vi "Raw Data to Scaled Data.vi"(8 "error In":errorcluster, 9 "Data":dbl[][](array[numeric]) caption="wfm" format="%.2f", 10 "Wvf Info":T1(array[cluster]) caption="wfm info" {"reserved2" format="%.2f"; "reserved1" format="%.2f"; "offset" format="%^.3e"; "gain" format="%^.3e"; "xIncrement" format="%^.3e"; "relativeInitialX" format="%^.3e"; "absoluteInitialX" format="%^.3e"}) -> (0 "error out":errorcluster, 1 "Scaled Current":dbl[](graph), 2 "Scaled Voltage":dbl[](graph), 4 "Raw Current":dbl[](graph), 5 "Raw Voltage":dbl[](graph))   [LabVIEW 2018]
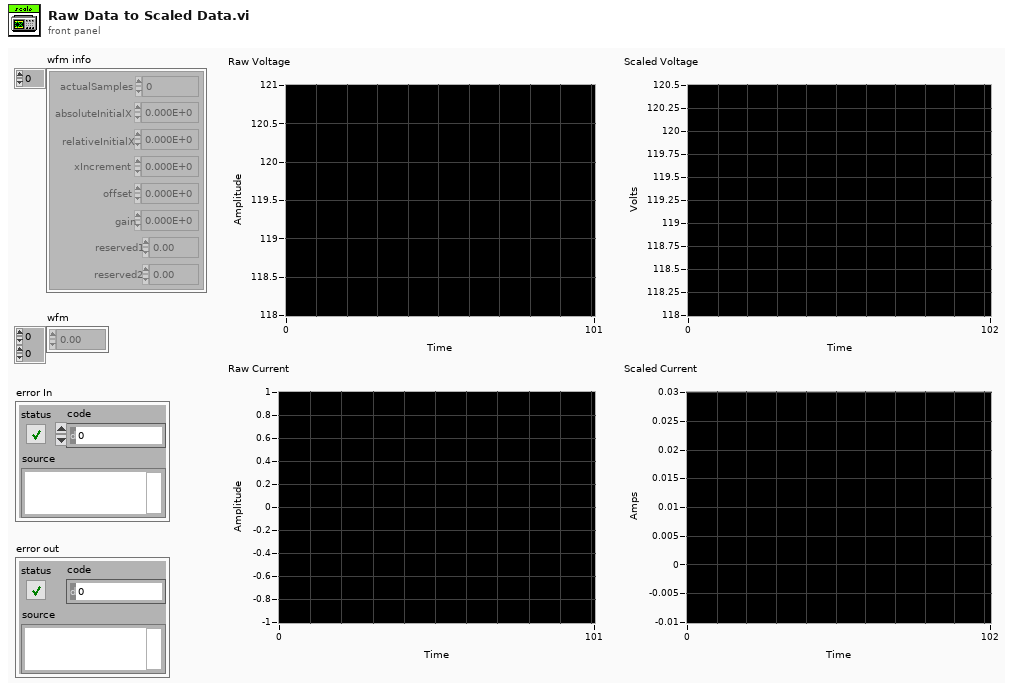
[diagram p1: front panel]
types:
  T1 = cluster{"actualSamples":i32, "absoluteInitialX":dbl, "relativeInitialX":dbl, "xIncrement":dbl, "offset":dbl, "gain":dbl, "reserved1":dbl, "reserved2":dbl}[]
  T2 = cluster{"actualSamples":i32, "absoluteInitialX":dbl, "relativeInitialX":dbl, "xIncrement":dbl, "offset":dbl, "gain":dbl, "reserved1":dbl, "reserved2":dbl}
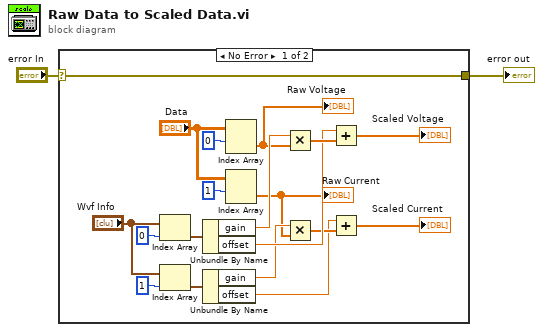
[diagram p0: block diagram]
diagram:
  n1 = case shown="No Error" "error In" {
    selector: "error In" -> [w5 w22]
    tunnel: [w5 w22] -> w1
    frame No Error {
      n2 = Index Array(array="Wvf Info", index=0) -> (element=w19:T2)
      n3 = Index Array(array="Wvf Info", index=1) -> (element=w13:T2)
      n4 = Unbundle By Name(w19) -> ("gain"=w17:dbl, "offset"=w16:dbl)
      n5 = Unbundle By Name(w13) -> ("gain"=w10:dbl, "offset"=w11:dbl)
      n6 = Index Array(array="Data", index (row)=0) -> (element=w6:dbl[])  [unwired: 1 in]
      "Raw Voltage" <- w6
      n7 = Index Array(array="Data", index (row)=1) -> (element=w7:dbl[])  [unwired: 1 in]
      "Raw Current" <- w7
      n8 = Multiply(x=w17, y=w6) -> (x*y=w18:dbl[])
      n9 = Multiply(x=w10, y=w7) -> (x*y=w12:dbl[])
      n10 = Add(x=w16, y=w18) -> (x+y=→"Scaled Voltage":dbl[])
      n11 = Add(x=w11, y=w12) -> (x+y=→"Scaled Current":dbl[])
    }
    frame Error {
    }
  }
  "error out" <- w1
